vi "SetValues.vi"(9 "error in":errorcluster) -> (1 "error out":errorcluster)   [LabVIEW 2017]
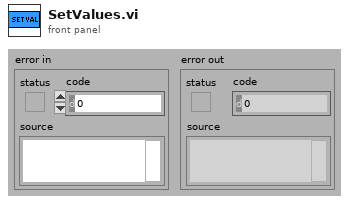
[diagram p1: front panel]
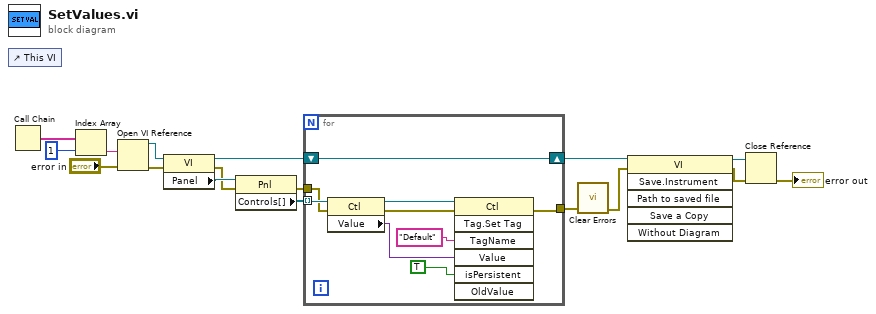
[diagram p0: block diagram]
diagram:
  n1 = control-ref of="This VI"() -> ()  [unwired: 1 out]
  n2 = Call Chain() -> (call chain=w17:string[])
  n3 = Index Array(array=w17, index=1) -> (element=w16:string)
  n4 = Open VI Reference(vi path=w16, error in (no error)="error in") -> (vi reference=w9:refnum<vi>, error out=w10:errorcluster)  [unwired: 4 in]
  n5 = property class="VI"(reference=w9, error in=w10) -> (reference out=w11:refnum<vi>, error out=w13:errorcluster, "Panel"=w14:refnum<vi>)
  n6 = property class="Pnl"(reference=w14, error in=w13) -> (error out=w8:errorcluster, "Controls[]"=w12:refnum<vi>[])  [unwired: 1 out]
  n7 = for {
    tunnel: w12 -> [w19] mode=indexing
    shift-right: [w26] -> w2
    shift-left: w11 -> [w26]
    tunnel: [w20] -> w6
    tunnel: w8 -> [w18]
    n8 = property class="Ctl"(reference=w19, error in=w18) -> (reference out=w23:refnum<vi>, error out=w25:errorcluster, "Value"=w24:variant)
    n9 = invoke class="Ctl" method="Tag.Set Tag"(reference=w23, error in=w25, "TagName"="Default" ("Tag Name"), "Value"=w24, "isPersistent"=TRUE ("Is Persistent?")) -> (error out=w20:errorcluster)  [unwired: 2 in, 6 out]
  }
  n10 = call <vilib>:"Clear Errors.vi"("error in (no error)"=w6) -> ("error out"=w3:errorcluster)  [unwired: 5 in, 1 out]
  n11 = invoke class="VI" method="Save.Instrument"(reference=w2, error in=w3) -> (reference out=w5:refnum<vi>, error out=w4:errorcluster)  [unwired: 4 in, 4 out]
  n12 = Close Reference(reference=w5, error in (no error)=w4) -> (error out=→"error out":errorcluster)
